vi "Get Active Tree.vi"(8 "error in (no error)":errorcluster, 11 "Tree in":refnum<class "Tree.lvclass">) -> (0 "error out":errorcluster, 2 "Returned tree out":refnum<class "Tree.lvclass">, 3 "Tree out":refnum<class "Tree.lvclass">)   [LabVIEW 2012, in "MDSplus.lvlib" / "Tree.lvclass"]
doc: "Returns the currently opened and active tree."
uses:
  <vilib>/MDSplus/Classes/Tree_Class/Tree.lvclass
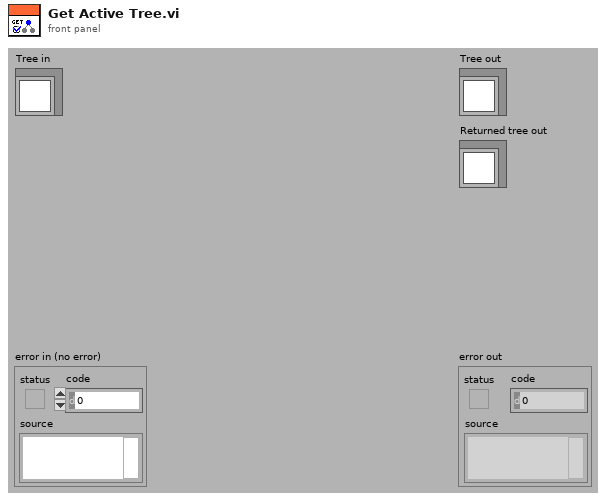
[diagram p1: front panel]
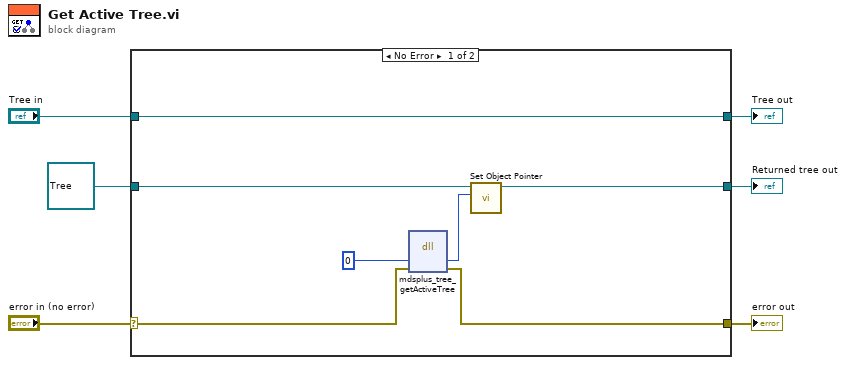
[diagram p0: block diagram]
diagram:
  n1 = case shown="No Error" "error in (no error)" {
    selector: "error in (no error)" -> [w9 w16]
    tunnel: [w8 w16] -> w5
    tunnel: [w11 w15] -> w3
    tunnel: refnum<class "Tree.lvclass"> refnum ("Tree in") -> [w12 w15]
    tunnel: [w7 w14] -> w2
    tunnel: "Tree in" -> [w7 w14]
    frame No Error {
      n2 = dll-call lib="MDSobjectsLVShr" fn="mdsplus_tree_getActiveTree"("lvTreePtrOut"=i64 0 ("lvTreePtr"), "error"=w9) -> ("lvTreePtrOut"=w10:i64, "error"=w8:errorcluster)  [unwired: 4 in, 2 out]
      n3 = call-dynamic "Set Object Pointer.vi"("Object Pointer"=w10, "Tree in"=w12) -> ("Tree out"=w11:refnum<class "Tree.lvclass">)  [unwired: 9 in]
    }
    frame Error {
    }
  }
  "error out" <- w5
  "Returned tree out" <- w3
  "Tree out" <- w2
